vi "Control Type.vi"(11 "LatchedValve in":refnum<class "LatchedValve.lvclass">) -> (2 "Valve Type":string)   [LabVIEW 2020, in "VolatusControl.lvlib" / "LatchedValve.lvclass"]
uses:
  LatchedValve.lvclass
  LatchedValve.lvclass/LatchedValve.ctl
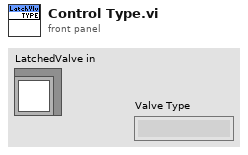
[diagram p1: front panel]
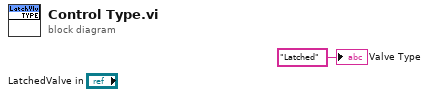
[diagram p0: block diagram]
diagram:
  "Valve Type" <- "Latched" ("Valve Type")
